vi "getVariableHeaderLength.vi"(11 "CONNECT in":refnum<class "CONNECT.lvclass">) -> (1 "size definitive":bool, 2 "VariableHeader size":u32, 3 "CONNECT out":refnum<class "CONNECT.lvclass">)   [LabVIEW 2013, in "CONNECT.lvclass"]
uses:
  CONNECT.lvclass
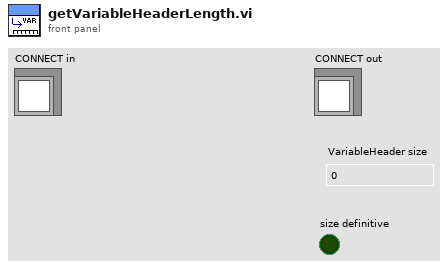
[diagram p1: front panel]
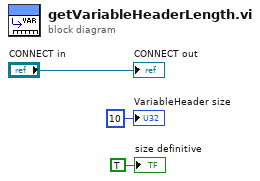
[diagram p0: block diagram]
diagram:
  "CONNECT out" <- "CONNECT in"
  "VariableHeader size" <- u32 10 ("VariableHeader size")
  "size definitive" <- TRUE ("size definitive")
